vi "HDLC_send_byte.vi"(10 "byte":u8 format="%x", 11 "VISA resource name":refnum<visa-resource-name>) -> ()   [LabVIEW 2018]
uses:
  special_characters.ctl
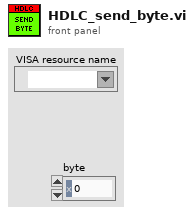
[diagram p1: front panel]
types:
  T1 = typedef "special_characters.ctl" = u8
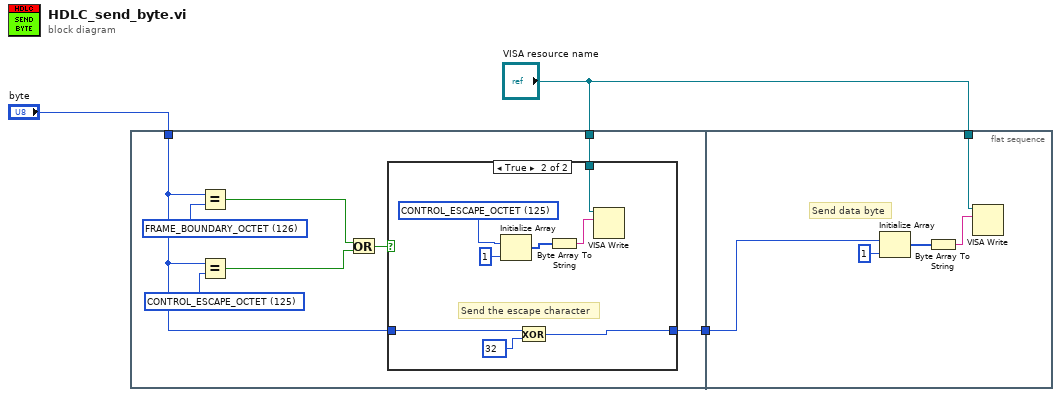
[diagram p0: block diagram]
diagram:
  n1 = flat-sequence {
    tunnel: "byte" -> [w5]
    tunnel: "VISA resource name" -> [w6]
    tunnel: [w4] -> w3
    tunnel: w3 -> [w23]
    tunnel: "VISA resource name" -> [w21]
    frame #0 {
      w10 = T1 125 items=["FRAME_BOUNDARY_OCTET"=126, "CONTROL_ESCAPE_OCTET"=125, "INVERT_OCTET"=32] ("Ring")
      w11 = T1 126 items=["FRAME_BOUNDARY_OCTET"=126, "CONTROL_ESCAPE_OCTET"=125, "INVERT_OCTET"=32] ("Ring")
      n2 = Equal?(x=w5, y=w11) -> (x = y?=w9:bool)
      n3 = Equal?(x=w5, y=w10) -> (x = y?=w8:bool)
      n4 = Or(x=w9, y=w8) -> (x .or. y?=w7:bool)
      n5 = case shown="True" w7 {
        tunnel: w6 -> [_ w20]
        tunnel: w5 -> [w12 w14]
        tunnel: [w12 w13] -> w4
        frame False {
        }
        frame True {
          w16 = T1 125 items=["FRAME_BOUNDARY_OCTET"=126, "CONTROL_ESCAPE_OCTET"=125, "INVERT_OCTET"=32] ("Ring")
          # "Send the escape character"
          n6 = Initialize Array(w16, 1 ("dimension size")) -> (w18:T1[])
          n7 = Exclusive Or(1:u8 32 ("y"), 2:w14) -> (0:w13:u8)
          n8 = Byte Array To String(unsigned byte array=w18) -> (string=w17:string)
          n9 = VISA Write(VISA resource name=w20, write buffer=w17) -> ()  [unwired: 1 in, 3 out]
        }
      }
    }
    frame #1 {
      # "Send data byte"
      n10 = Initialize Array(w23, 1 ("dimension size")) -> (w22:u8[])
      n11 = Byte Array To String(unsigned byte array=w22) -> (string=w24:string)
      n12 = VISA Write(VISA resource name=w21, write buffer=w24) -> ()  [unwired: 1 in, 3 out]
    }
  }
